vi "Read App Ref.vi"(11 "Base Attributes in":refnum<class "Base Attributes.lvclass">) -> (2 "App Ref":refnum<vi>)   [LabVIEW 2020, in "jettl.lvlib" / "Base Attributes.lvlib" / "Base Attributes.lvclass"]
uses:
  Base Attributes.lvclass
  Base Attributes.lvclass/Base Attributes.ctl
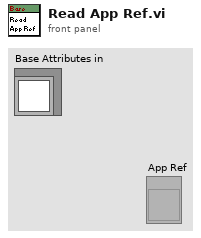
[diagram p1: front panel]
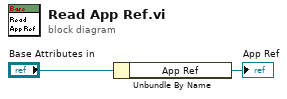
[diagram p0: block diagram]
diagram:
  n1 = Unbundle By Name("Base Attributes in") -> ("App Ref"=→"App Ref":refnum<vi>)
